vi "Test Waveform Components (SubVI).vi"(10 "Y position":dbl, 11 "Power Spectrum":dynamicdata(waveform)) -> (1 "waveform out":waveform(dbl), 2 "X value":timestamp, 3 "Array of Waveform":waveform(dbl)[](array[waveform]), 4 "actual Y position":dbl, 5 "Y value":dbl)   [LabVIEW 2021]
uses:
  <vilib>/Waveform/WDTOps.llb/WDT Get XY Value DBL.vi
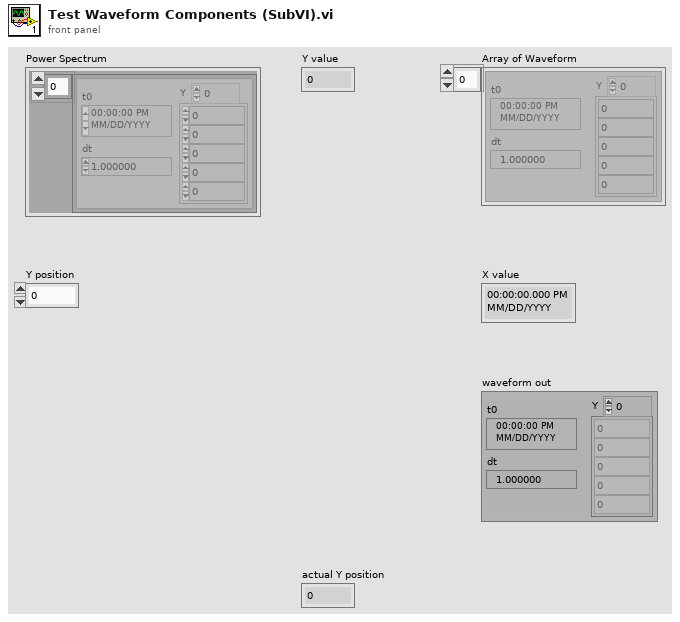
[diagram p1: front panel]
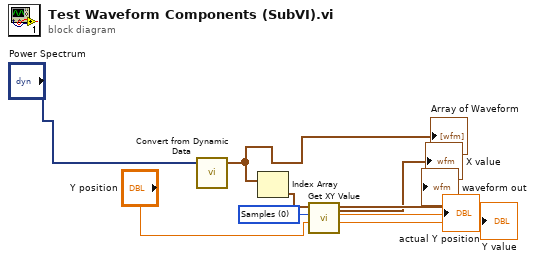
[diagram p0: block diagram]
diagram:
  w5 = u16 0 items=["Samples", "Relative Time"] ("Y position format")
  n1 = call "Convert from Dynamic Data"("Dynamic Data Type"="Power Spectrum") -> ("Array of Waveform"=w2:waveform(dbl)[])  [unwired: 3 in]
  "Array of Waveform" <- w2
  n2 = Index Array(array=w2) -> (element=w3:waveform(dbl))  [unwired: 1 in]
  n3 = call-poly <vilib>:"Get XY Value.vi"("Y position"="Y position", "Y position format"=w5, "waveform in"=w3) -> ("Y value"=→"Y value":dbl, "actual Y position"=→"actual Y position":dbl, "waveform out"=→"waveform out":waveform(dbl), "X value"=→"X value":timestamp)  [unwired: 4 in, 1 out]
